vi "Scada_MezclarColores.vi"() -> ()   [LabVIEW 2020]
uses:
  VariablesGlobales.vi
panel:
  out "Contador de Galones":dbl
  out "LSL 5":bool
  out "LSL 4":bool
  out "LSL 3":bool
  out "LSL 2":bool
  out "LSL 1":bool
  out "LSH 5":bool
  out "LSH 4":bool
  out "LSH 3":bool
  out "LSH 2":bool
  out "LSH 1":bool
  out "M1":bool
  out "FV 5":bool
  out "FV 4":bool
  out "FV 3":bool
  out "FV 2":bool
  out "FV 1":bool
  out "Mixer":bool
  out "Galón":bool
  out "Cilindro 2":bool
  out "Sellado":bool
  out "S 9":bool
  out "S 8":bool
  out "S 7":bool
  out "S 6":bool
  out "S 5":bool
  out "S 4":bool
  out "S 3":bool
  out "S 2":bool
  out "S 1":bool
  out "FIT 1":dbl
  out "B 5":bool
  out "B 4":bool
  out "B 3":bool
  out "B 2":bool
  out "B 1":bool
  out "FIT 5":dbl
  out "FIT 4":dbl
  out "FIT 3":dbl
  out "FIT 2":dbl
  out "tk blanco":dbl(slide) scale=0.0..100.0
  out "tk negro":dbl(slide) scale=0.0..100.0
  out "tk azul":dbl(slide) scale=0.0..100.0
  out "tk amarillo":dbl(slide) scale=0.0..100.0
  out "tk rojo":dbl(slide) scale=0.0..100.0
  in  "Panel_Color":T1
  # "Yellow"
  # "Red"
  # "Blue"
  # "Black"
  # "White"
  # "gal"
  # "gal"
  # "gal"
  # "gal"
  # "gal"
  # "Etiquetado"
  # "Mezclado"
  # "gal"
  # "gal"
  # "gal"
  # "gal"
  # "Unidades"
  # "FV 1"
  # "FV 2"
  # "FV 3"
  # "FV 4"
  # "FV 5"
  # "gal"
  # "Panel de Selección de Color"
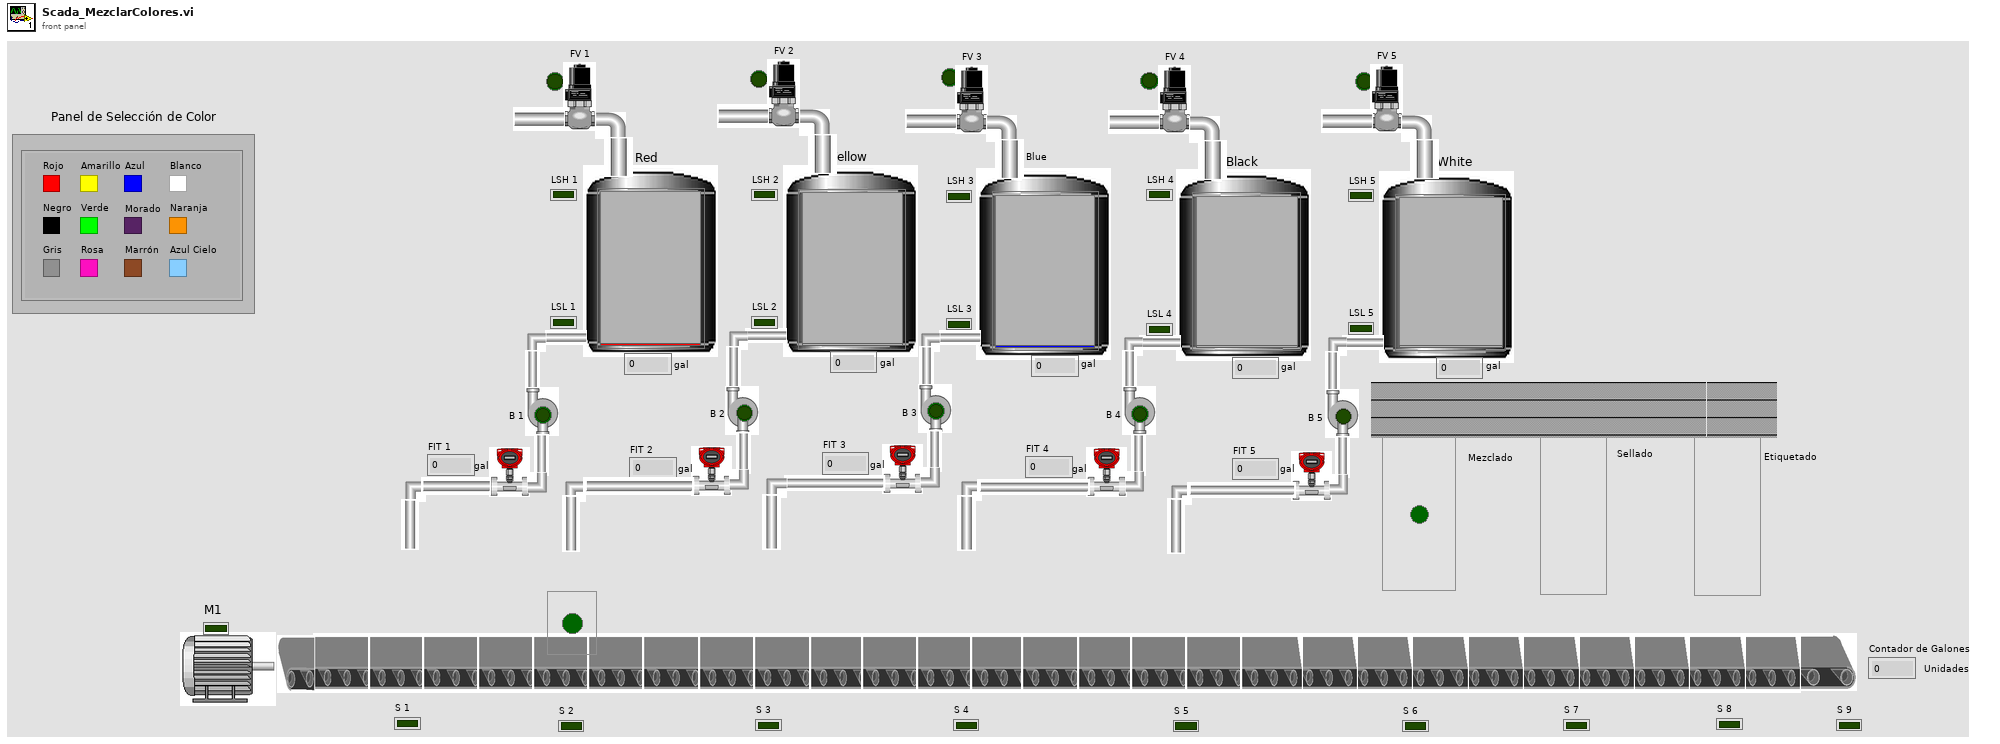
[diagram p1: front panel]
types:
  T1 = cluster{"Rojo":bool, "Amarillo":bool, "Azul":bool, "Blanco":bool, "Negro":bool, "Verde":bool, "Morado":bool, "Naranja":bool, "Gris":bool, "Rosa":bool, "Marrón ":bool, "Azul Cielo":bool}
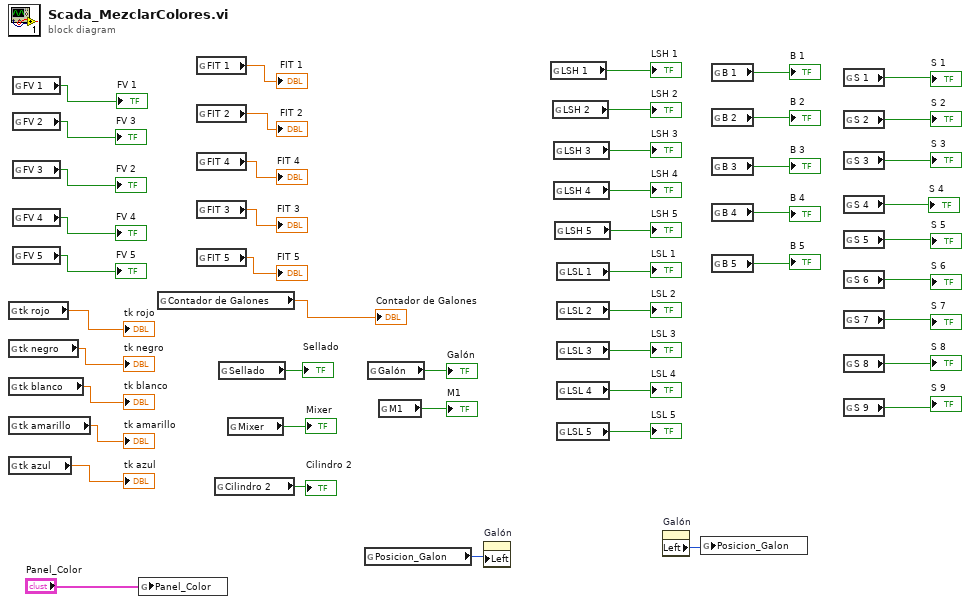
[diagram p0: block diagram]
diagram:
  n1 = global read "VariablesGlobales.vi" "tk rojo"() -> (→"tk rojo":dbl)
  n2 = global read "VariablesGlobales.vi" "tk negro"() -> (→"tk negro":dbl)
  n3 = global read "VariablesGlobales.vi" "tk blanco"() -> (→"tk blanco":dbl)
  n4 = global read "VariablesGlobales.vi" "tk amarillo"() -> (→"tk amarillo":dbl)
  n5 = global read "VariablesGlobales.vi" "tk azul"() -> (→"tk azul":dbl)
  n6 = global read "VariablesGlobales.vi" "FV 1"() -> (→"FV 1":bool)
  n7 = global read "VariablesGlobales.vi" "FV 2"() -> (→"FV 3":bool)
  n8 = global read "VariablesGlobales.vi" "FV 3"() -> (→"FV 2":bool)
  n9 = global read "VariablesGlobales.vi" "FV 4"() -> (→"FV 4":bool)
  n10 = global read "VariablesGlobales.vi" "FV 5"() -> (→"FV 5":bool)
  n11 = global write "VariablesGlobales.vi" "Panel_Color"("Panel_Color") -> ()
  n12 = global read "VariablesGlobales.vi" "Contador de Galones"() -> (→"Contador de Galones":dbl)
  n13 = global read "VariablesGlobales.vi" "FIT 1"() -> (→"FIT 1":dbl)
  n14 = global read "VariablesGlobales.vi" "FIT 2"() -> (→"FIT 2":dbl)
  n15 = global read "VariablesGlobales.vi" "FIT 4"() -> (→"FIT 4":dbl)
  n16 = global read "VariablesGlobales.vi" "FIT 3"() -> (→"FIT 3":dbl)
  n17 = global read "VariablesGlobales.vi" "FIT 5"() -> (→"FIT 5":dbl)
  n18 = global read "VariablesGlobales.vi" "Cilindro 2"() -> (→"Cilindro 2":bool)
  n19 = global read "VariablesGlobales.vi" "Sellado"() -> (→"Sellado":bool)
  n20 = global read "VariablesGlobales.vi" "Mixer"() -> (→"Mixer":bool)
  n21 = global read "VariablesGlobales.vi" "Posicion_Galon"() -> (w3:i32)
  n22 = global read "VariablesGlobales.vi" "Galón"() -> (→"Galón":bool)
  n23 = global read "VariablesGlobales.vi" "M1"() -> (→"M1":bool)
  n24 = property on="Galón" class="Bool (strict)"("Left"=w3) -> ()  [unwired: 2 in, 2 out]
  n25 = global read "VariablesGlobales.vi" "LSH 1"() -> (→"LSH 1":bool)
  n26 = global read "VariablesGlobales.vi" "LSH 2"() -> (→"LSH 2":bool)
  n27 = global read "VariablesGlobales.vi" "LSH 3"() -> (→"LSH 3":bool)
  n28 = global read "VariablesGlobales.vi" "LSH 4"() -> (→"LSH 4":bool)
  n29 = global read "VariablesGlobales.vi" "LSH 5"() -> (→"LSH 5":bool)
  n30 = global read "VariablesGlobales.vi" "LSL 1"() -> (→"LSL 1":bool)
  n31 = global read "VariablesGlobales.vi" "LSL 2"() -> (→"LSL 2":bool)
  n32 = global read "VariablesGlobales.vi" "LSL 3"() -> (→"LSL 3":bool)
  n33 = global read "VariablesGlobales.vi" "LSL 4"() -> (→"LSL 4":bool)
  n34 = global read "VariablesGlobales.vi" "LSL 5"() -> (→"LSL 5":bool)
  n35 = property on="Galón" class="Bool (strict)"() -> ("Left"=w2:i32)  [unwired: 2 in, 2 out]
  n36 = global write "VariablesGlobales.vi" "Posicion_Galon"(w2) -> ()
  n37 = global read "VariablesGlobales.vi" "B 1"() -> (→"B 1":bool)
  n38 = global read "VariablesGlobales.vi" "B 2"() -> (→"B 2":bool)
  n39 = global read "VariablesGlobales.vi" "B 3"() -> (→"B 3":bool)
  n40 = global read "VariablesGlobales.vi" "B 4"() -> (→"B 4":bool)
  n41 = global read "VariablesGlobales.vi" "B 5"() -> (→"B 5":bool)
  n42 = global read "VariablesGlobales.vi" "S 1"() -> (→"S 1":bool)
  n43 = global read "VariablesGlobales.vi" "S 2"() -> (→"S 2":bool)
  n44 = global read "VariablesGlobales.vi" "S 3"() -> (→"S 3":bool)
  n45 = global read "VariablesGlobales.vi" "S 4"() -> (→"S 4":bool)
  n46 = global read "VariablesGlobales.vi" "S 5"() -> (→"S 5":bool)
  n47 = global read "VariablesGlobales.vi" "S 6"() -> (→"S 6":bool)
  n48 = global read "VariablesGlobales.vi" "S 7"() -> (→"S 7":bool)
  n49 = global read "VariablesGlobales.vi" "S 8"() -> (→"S 8":bool)
  n50 = global read "VariablesGlobales.vi" "S 9"() -> (→"S 9":bool)
